vi "GetDriveQueue.vi"(8 "error in (no error)":errorcluster) -> (0 "error out":errorcluster, 3 "queue out":refnum<queue>)   [LabVIEW 2013]
doc: "Outputs the drive queue (of type DriveQueueInstruction), and opens it if necessary (i.e. in Begin)."
uses:
  DriveInstruction.ctl
  DriveData.ctl
  QueueSubsystem.ctl
  TankDriveAction.ctl
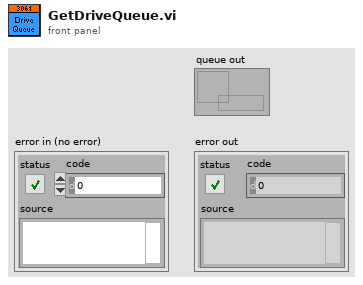
[diagram p1: front panel]
types:
  T1 = typedef "DriveInstruction.ctl" = cluster{"DriveData":T2, "Subsystem":T3, "Action":T4}
  T2 = typedef "DriveData.ctl" = cluster{"cDriveLeft":dbl, "cDriveRight":dbl, "cHalfDrive":bool, "cStraightDrive":bool, "cReverseDrive":bool}
  T3 = typedef "QueueSubsystem.ctl" = enum16{"Drive", "SonicShifter", "Kicker", "FiringPneumatic", "RollerPneumatic", "Clapper", "RollerMotor", "CollectorMotor"}
  T4 = typedef "TankDriveAction.ctl" = enum16{"Init", "LinearDrive", "SetValue", "Disable"}
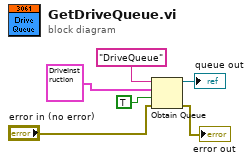
[diagram p0: block diagram]
diagram:
  n1 = Obtain Queue(name (unnamed)="DriveQueue", element data type=T1 {"DriveData"={"cDriveLeft"=0.0, "cDriveRight"=1.0, "cHalfDrive"=FALSE, "cStraightDrive"=FALSE, "cReverseDrive"=FALSE}, "Subsystem"=enum."SonicShifter", "Action"=enum."Init"} ("Cluster"), create if not found? (T)=TRUE, error in (no error)="error in (no error)") -> (queue out=→"queue out":refnum<queue>, error out=→"error out":errorcluster)  [unwired: 1 in, 1 out]
